vi "探头通信模块.vi"(11 "探头属性":T8={"探头地址与信息"={"网络地址"="四渡赤水", "名称"="四渡赤水", "备注"="10.10.100.254", "累积剂量"=8899.0, "累积限值"=0.0, "硬件剂量率限值"=enum."一级限值", "剂量率限值1"=0.0, "剂量率限值2"=0.0, "报警方式"=enum."常报警"}, "测量值"={"时间"=timestamp(0 s since 1904-01-01), "数值"=0.0}, "限值"={"限值1"=1.0, "限值2"=100.0, "探头限值"=enum."一级限值"}, "探头状态"=enum."离线", "累积记录"={"起始时间"=timestamp(0 s since 1904-01-01), "结束时间"=timestamp(0 s since 1904-01-01), "累积剂量"=0.0}, "报警方式"={"报警方式"=enum."常报警", "延迟计时"=0, "报警中？"=FALSE}}) -> ()   [LabVIEW 2017]
doc: "独立的探头TCP连接的接收处理模块，具有\"创建TCP连接\"，“自动同步报警限值”，“掉线重连”，“解析实时数据与报警数据”的功能。"
uses:
  <vilib>/Platform/TimedLoop/XDataNode/timing_clust.ctl
  <vilib>/Platform/TimedLoop/XDataNode/nitl_modes.ctl
  <vilib>/Platform/TimedLoop/XDataNode/wakeup.ctl
  0d55e998-beb3-44e2-a108-1cc669182013.vi
  <vilib>/regexp/Match Regular Expression.xnode
  <vilib>/Platform/TimedLoop/XDataNode/XDataNode.xnode
  <vilib>/Platform/TimedLoop/XDataNode/XDNodeRunTimeDep.lvlib
panel:
  in  "报警缓存防抖计次":i32
  in  "串口丢包次数":i32
  out "接收数据":string
  out "循环次数":i32
  out "TCP连接ID":refnum<k5>
  in  "通信错误":errorcluster caption="错误输出"
  in  "缓存结果":T1
  in  "改动项":T3
  in  "停止":bool
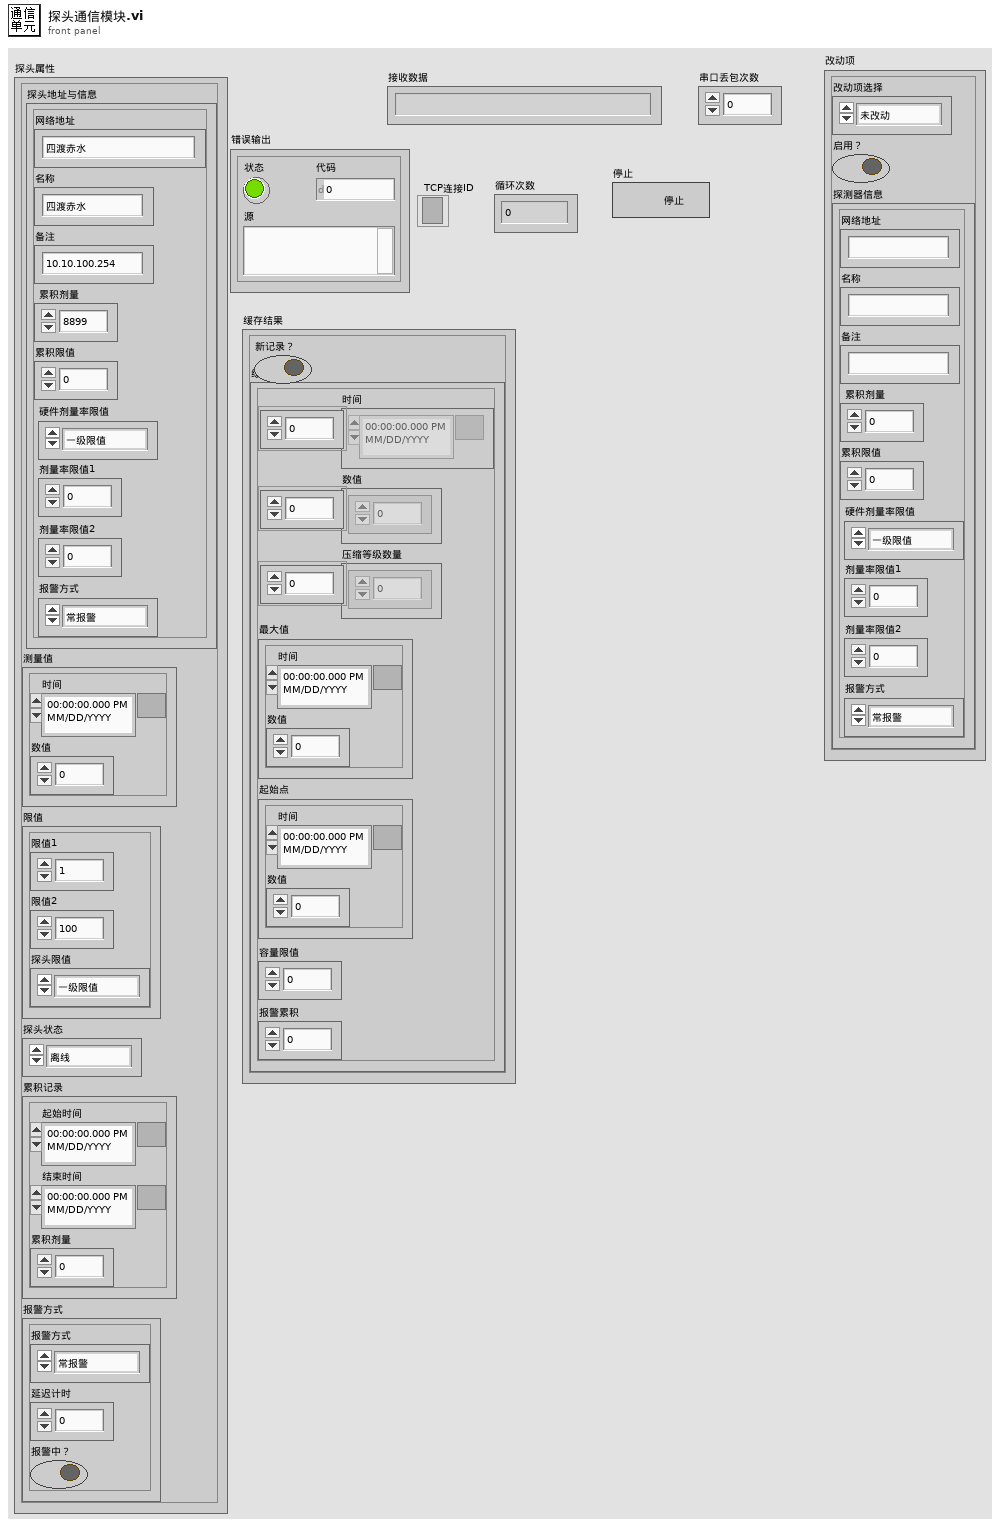
[diagram p1: front panel]
types:
  T1 = typedef "报警缓存状态与数据.ctl" = cluster{"新记录？":bool, "缓存数据":T2}
  T2 = typedef "时值缓存压缩模块.lvlib/缓存数据.ctl" = cluster{"时间":timestamp[], "数值":dbl[], "压缩等级数量":i32[], "最大值":cluster{"时间":timestamp, "数值":dbl}, "起始点":cluster{"时间":timestamp, "数值":dbl}, "容量限值":i32, "报警累积":dbl}
  T3 = typedef "改动项.ctl" = cluster{"改动项选择":T4, "启用？":bool, "探测器信息":T5}
  T4 = typedef "改动项选择.ctl" = enum16{"未改动", "改动-启用状态", "改动-探头信息", "改动-报警限值", "动作-手动静音", "动作-重启累积时段", "动作-累积删除", "动作-重连"}
  T5 = typedef "探测器信息.ctl" = cluster{"网络地址":string, "名称":string, "备注":string, "累积剂量":dbl, "累积限值":dbl, "硬件剂量率限值":T6, "剂量率限值1":dbl, "剂量率限值2":dbl, "报警方式":T7}
  T6 = typedef "探头剂量率限值选择.ctl" = enum16{"一级限值", "二级限值"}
  T7 = typedef "报警方式选择.ctl" = enum16{"常报警", "自动静音", "手动静音"}
  T8 = typedef "探头属性.ctl" = cluster{"探头地址与信息":T5, "测量值":T9, "限值":T10, "探头状态":T11, "累积记录":T12, "报警方式":T13}
  T9 = typedef "测量值.ctl" = cluster{"时间":timestamp, "数值":dbl}
  T10 = typedef "剂量率限值.ctl" = cluster{"限值1":dbl, "限值2":dbl, "探头限值":T6}
  T11 = typedef "探头状态.ctl" = enum16{"正常", "离线", "禁用", "一级报警", "二级报警", "累积报警"}
  T12 = typedef "单条累积记录.ctl" = cluster{"起始时间":timestamp, "结束时间":timestamp, "累积剂量":dbl}
  T13 = typedef "报警方式.ctl" = cluster{"报警方式":T7, "延迟计时":u16, "报警中？":bool}
  T14 = typedef "簇-输入.ctl" = cluster{"配置文件动作":T15, "数据输入":variant}
  T15 = typedef "枚举-配置文件动作.ctl" = enum16{"初始化加载配置", "读取配置", "写入-屏幕键盘", "写入-静音延迟", "写入-主要探头类型", "写入-串口配置", "写入-累积定时", "写入-导出定时", "保存配置到文件"}
  T16 = typedef "簇-配置文件内容.ctl" = cluster{"调试模式？":bool, "屏幕键盘？":bool, "软件版本":string, "静音延迟 s":u16, "主要探头类型":T17, "串口配置":cluster{"COM口":refnum<visa-resource-name>, "波特率":enum16{"9600", "19200"}, "读写超时ms":i16, "丢包判定次数":i16}, "定时配置-累积分段":T18, "定时配置-自动导出":cluster{"定时配置-自动导出":T18, "分别导出?":bool}}
  T17 = typedef "枚举-主要探头类型.ctl" = enum16{"网络探头", "串口探头"}
  T18 = typedef "簇-定时配置.ctl" = cluster{"定时模式":enum16{"绝对时间", "相对时间"}, "单位":enum16{"年", "月", "日", "时", "分"}, "间隔":u8, "目标时刻":timestamp}
  T19 = typedef "串口配置.ctl" = cluster{"COM口":refnum<visa-resource-name>, "波特率":enum16{"9600", "19200"}, "探头地址(U8)":u8}
  T20 = typedef "串口模块输入.ctl" = cluster{"串口动作类型":T21, "串口配置":T19, "数据输入":variant}
  T21 = typedef "串口动作类型.ctl" = enum16{"读测量值", "设置报警值", "设置地址", "设置系数", "广播修改波特率", "关闭串口"}
  T22 = typedef "DB动作与数据.ctl" = cluster{"动作类型":T23, "输入数据":variant}
  T23 = typedef "DB动作类型.ctl" = enum16{"DB-文件初始化+连接", "DB-断开连接", "DB-结构初始化", "DB-加载设备", "DB-检查连接状态", "设备-登记新设备+数据表", "设备-删除设备", "设备-修改网址", "设备-修改名称+转移数据", "设备-修改备注", "设备-修改限值", "设备-累积校准", "设备-重排", "数据-获取全部", "数据-删除数据", "数据-写改累积记录+改累积剂量", "读变量-全部设备"}
  T24 = typedef "测量值读取.ctl" = cluster{"测量值":dbl, "CRC":bool, "接收指令":string}
  T25 = typedef "写改累积记录输入.ctl" = cluster{"探头地址与信息":T5, "测量值":T9, "累积记录":T12}
  T26 = cluster{"报警方式":enum16{"常报警", "自动静音", "手动静音"}, "延迟计时":u16, "报警中？":bool}
  T27 = typedef "XDNodeRunTimeDep.lvlib/timing_clust.ctl" = cluster{"Expected End [f-1]":u64, "Actual End [f-1]":u64, "Finished Late? [f-1]":bool, "Expected End [i-1]":u64, "Actual End [i-1]":u64, "Finished Late? [i-1]":bool, "Expected Start [i]":u64, "Actual Start [i]":u64, "Expected Start [f]":u64, "Actual Start [f]":u64, "Source Name":string, "Structure Name":string, "Period":i64, "Deadline":i64, "Offset":i64, "Start":i64, "Priority":i32, "Timeout":i32, "Mode":T28, "Wakeup Reason":T29, "Error":errorcluster, "Source Type":string, "Secondary Source Type":string, "Global End Time":u64, "Global Start Time":u64, "Frame Duration":u64, "Iteration Duration":u64, "Assigned CPU":i32, "I/O Scan Engine Mode":u32}
  T28 = typedef "XDNodeRunTimeDep.lvlib/nitl_modes.ctl" = enum32{"No Change", "Process missed periods, maintain original phase", "Discard missed periods, maintain original phase", "Process missed periods, ignore original phase", "Discard missed periods, ignore original phase"}
  T29 = typedef "XDNodeRunTimeDep.lvlib/wakeup.ctl" = enum32{"Normal", "Aborted", "Asynchronous wakeup", "Timing source error", "Timed loop error", "Timeout"}
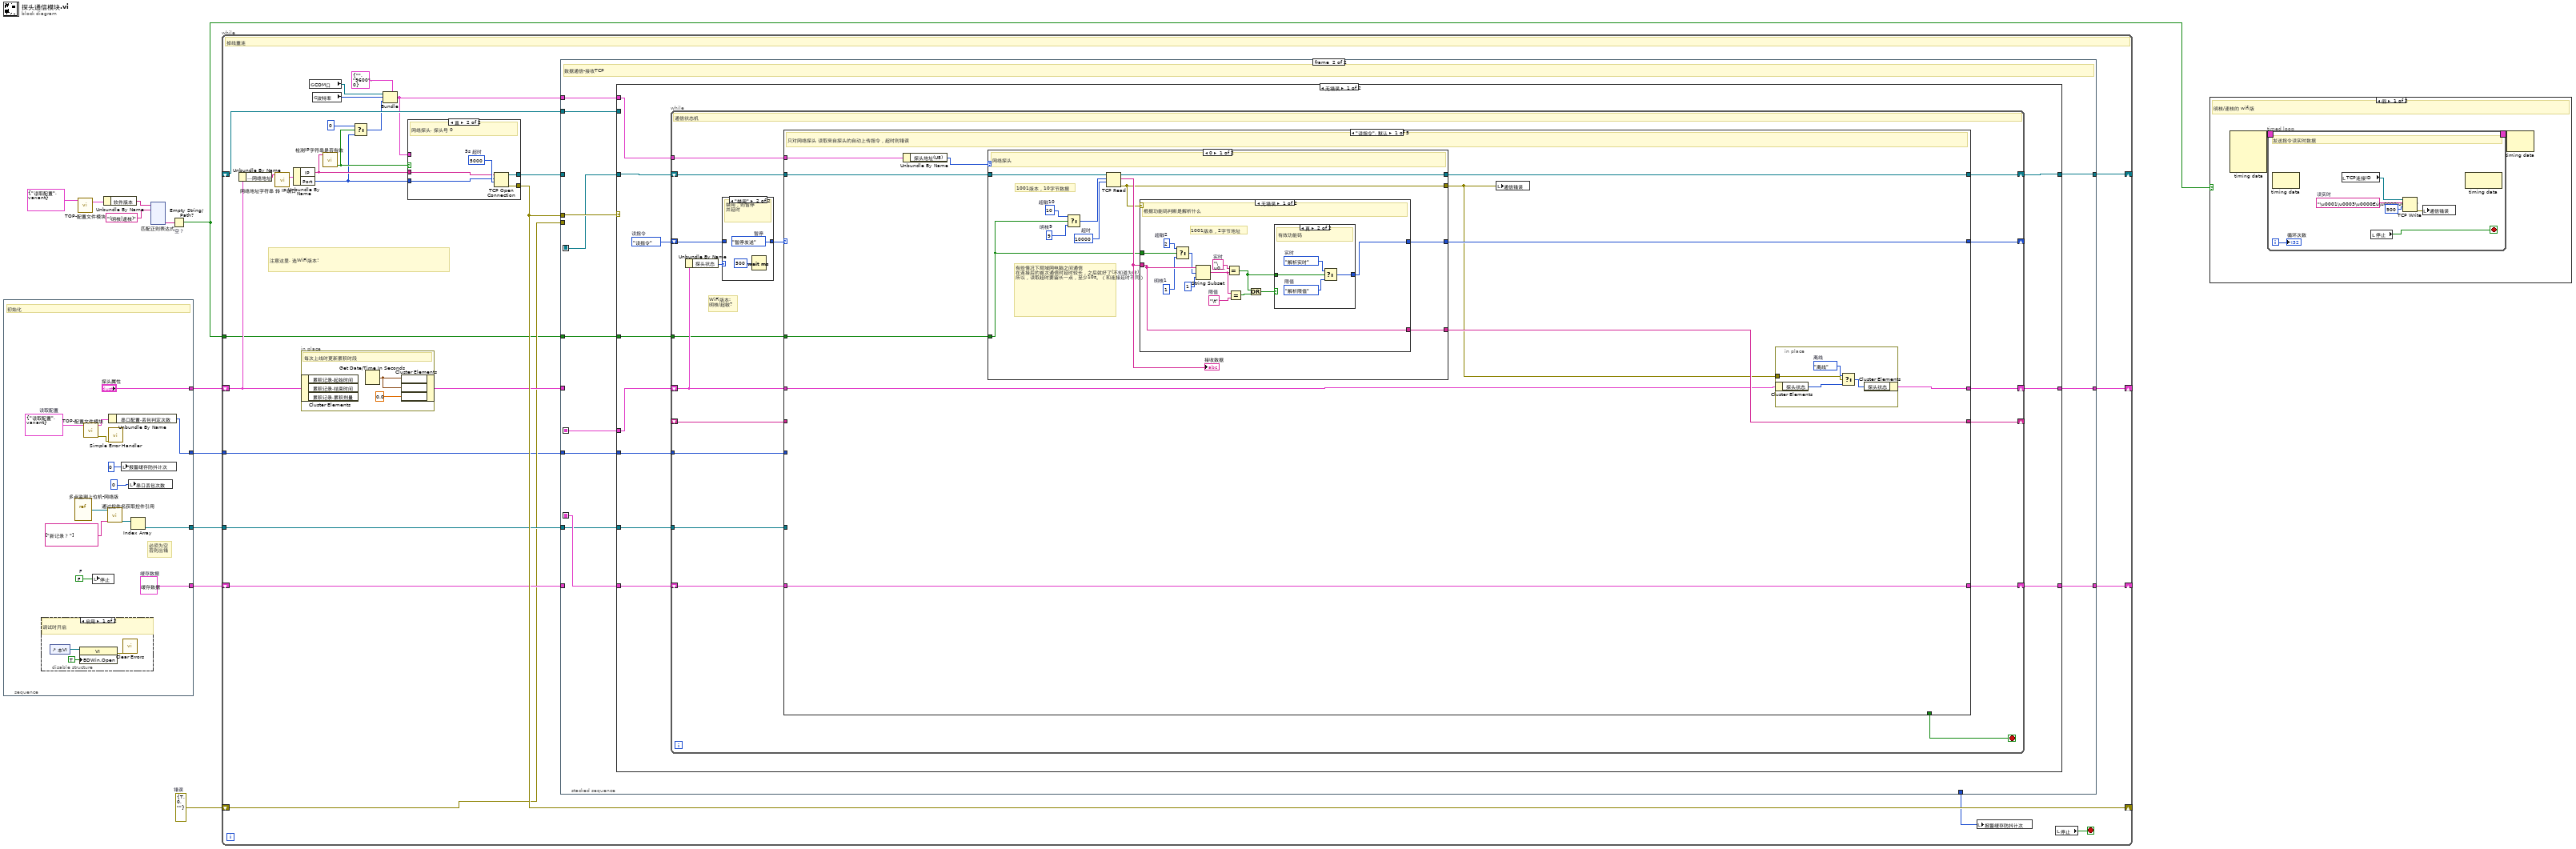
[diagram p0: block diagram]
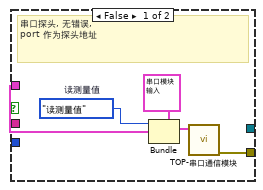
[diagram p4: hidden frame]
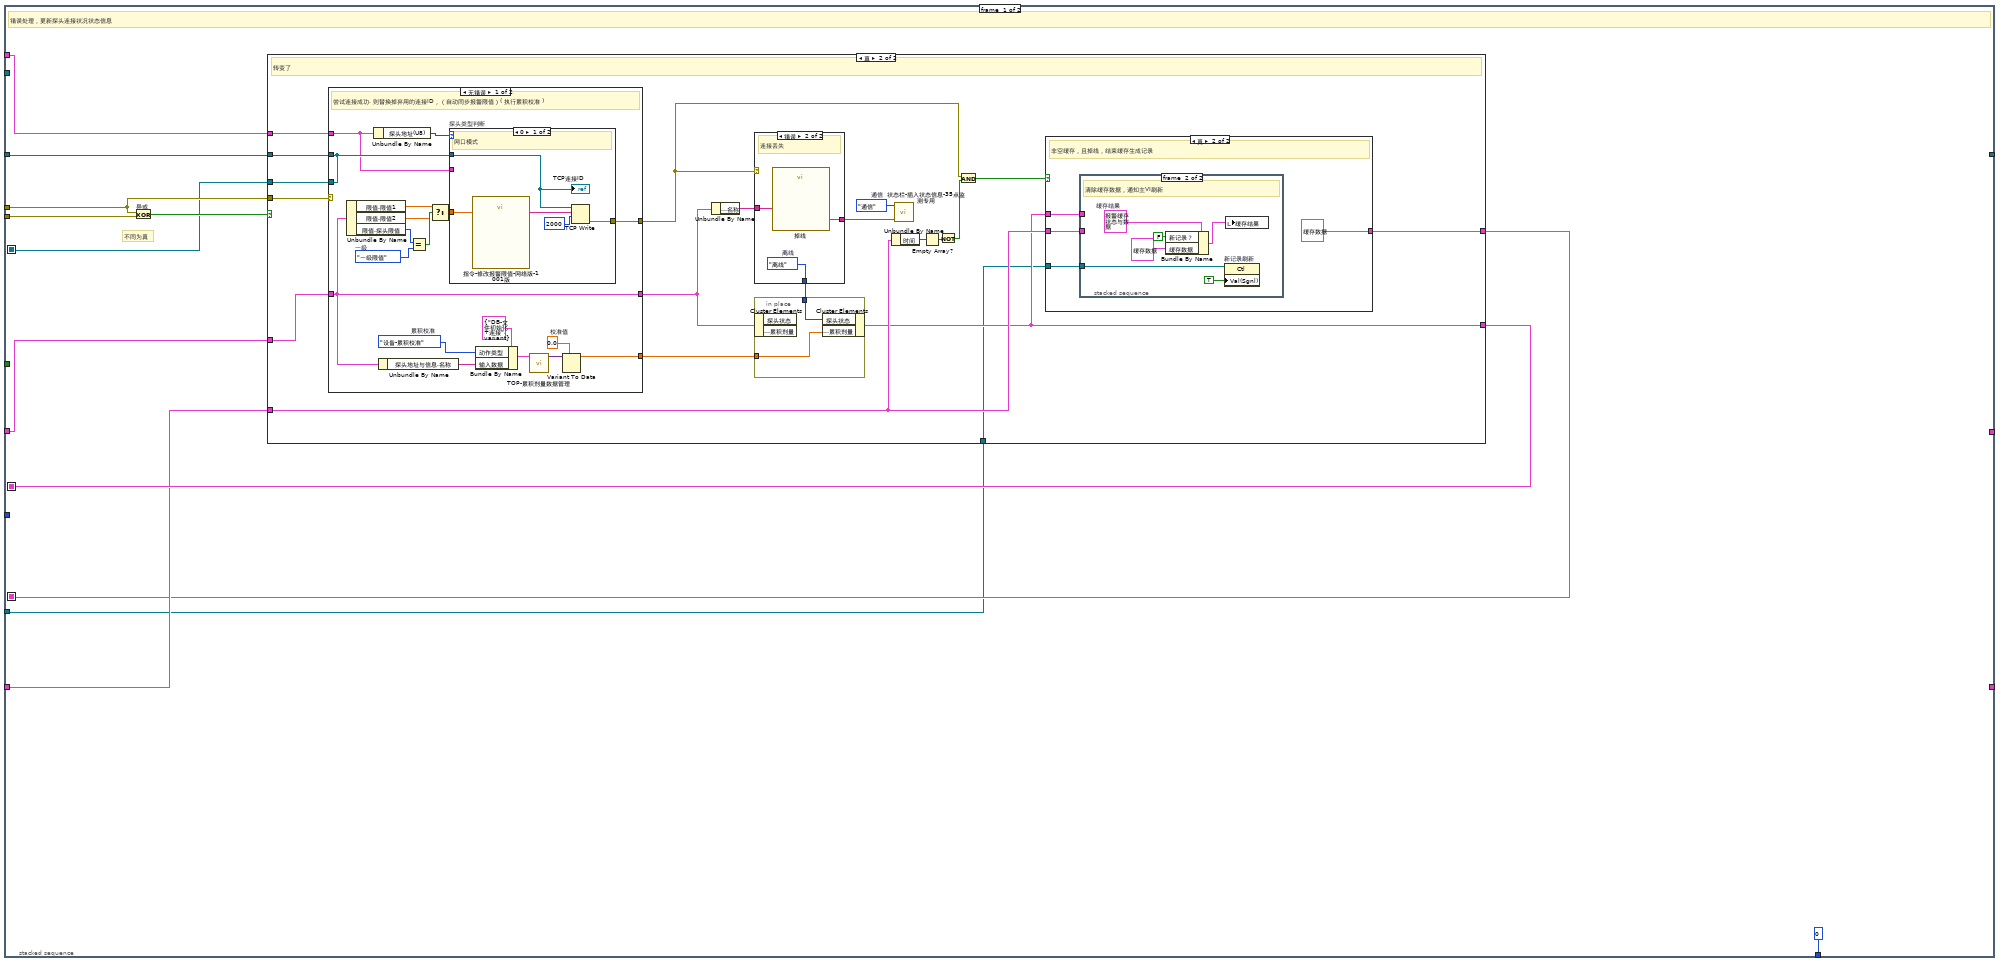
[diagram p5: hidden frame]
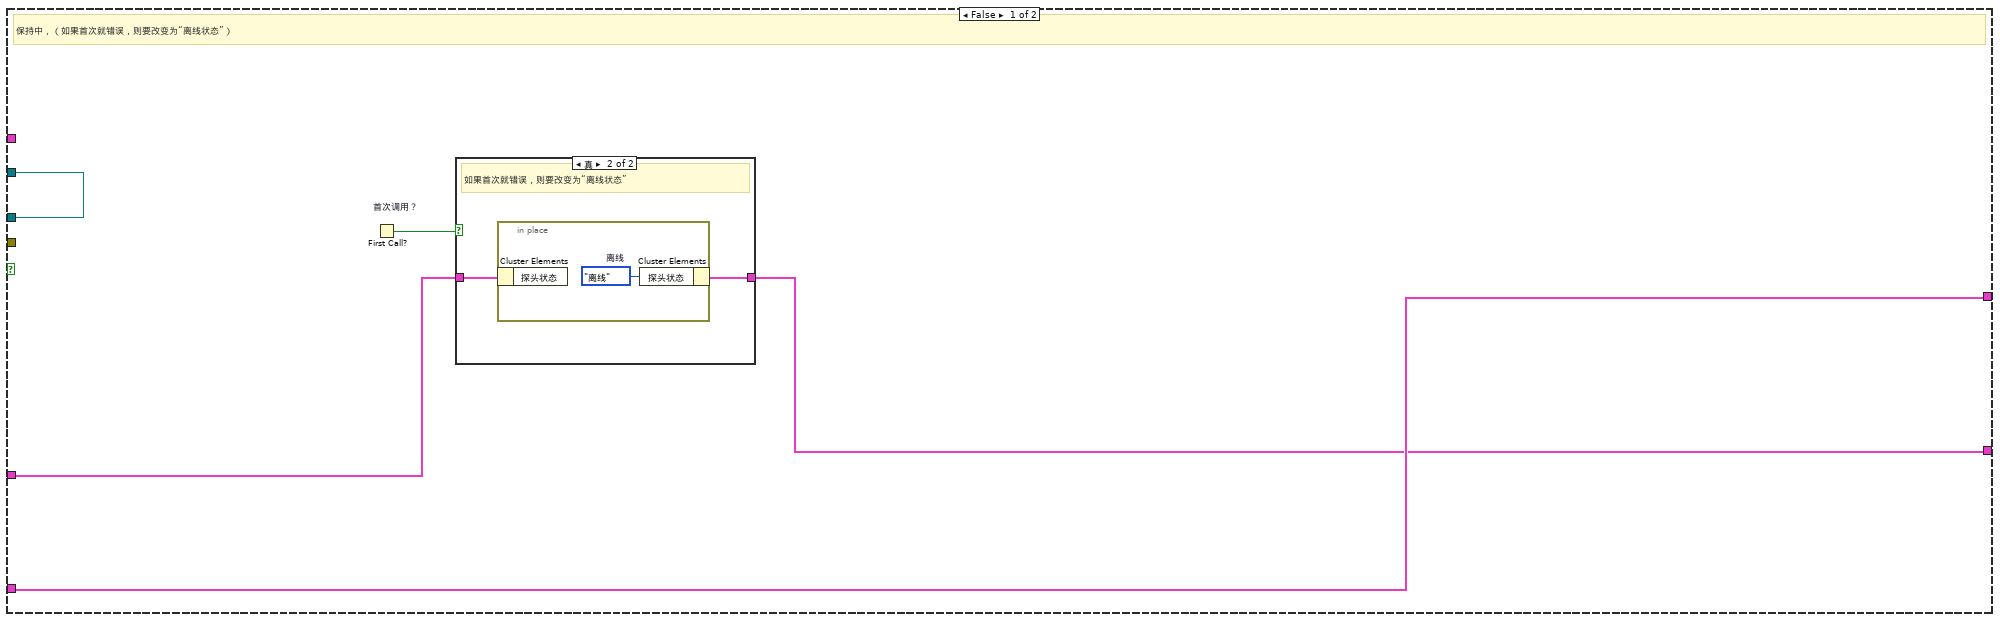
[diagram p6: hidden frame]
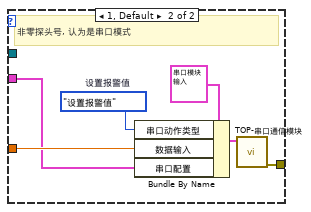
[diagram p8: hidden frame]
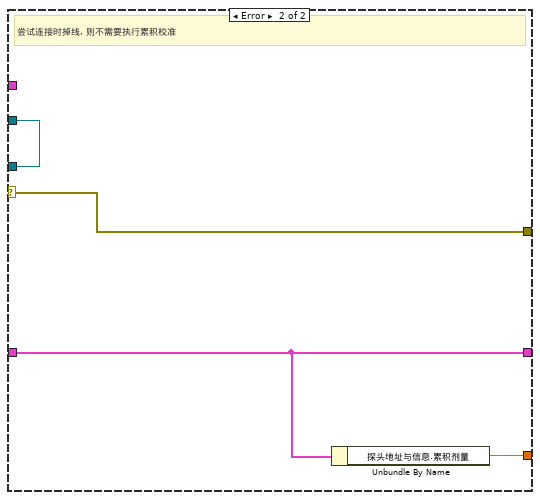
[diagram p9: hidden frame]
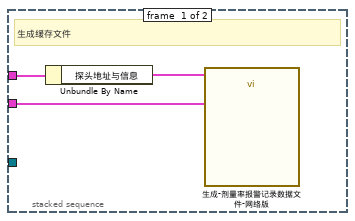
[diagram p11: hidden frame]
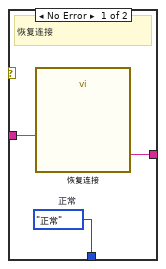
[diagram p12: hidden frame]
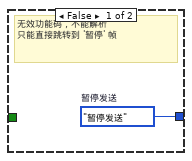
[diagram p14: hidden frame]
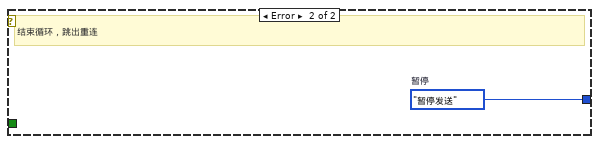
[diagram p15: hidden frame]
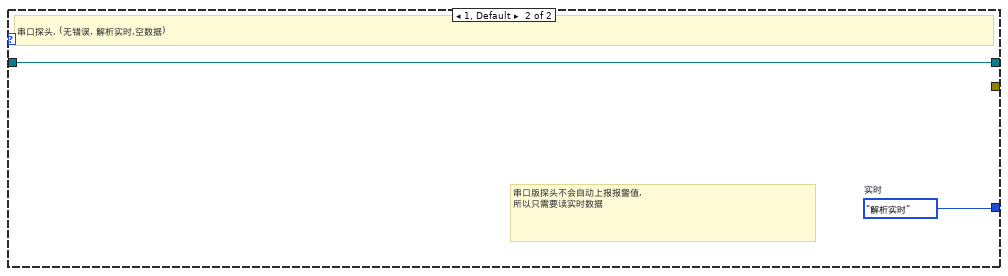
[diagram p16: hidden frame]
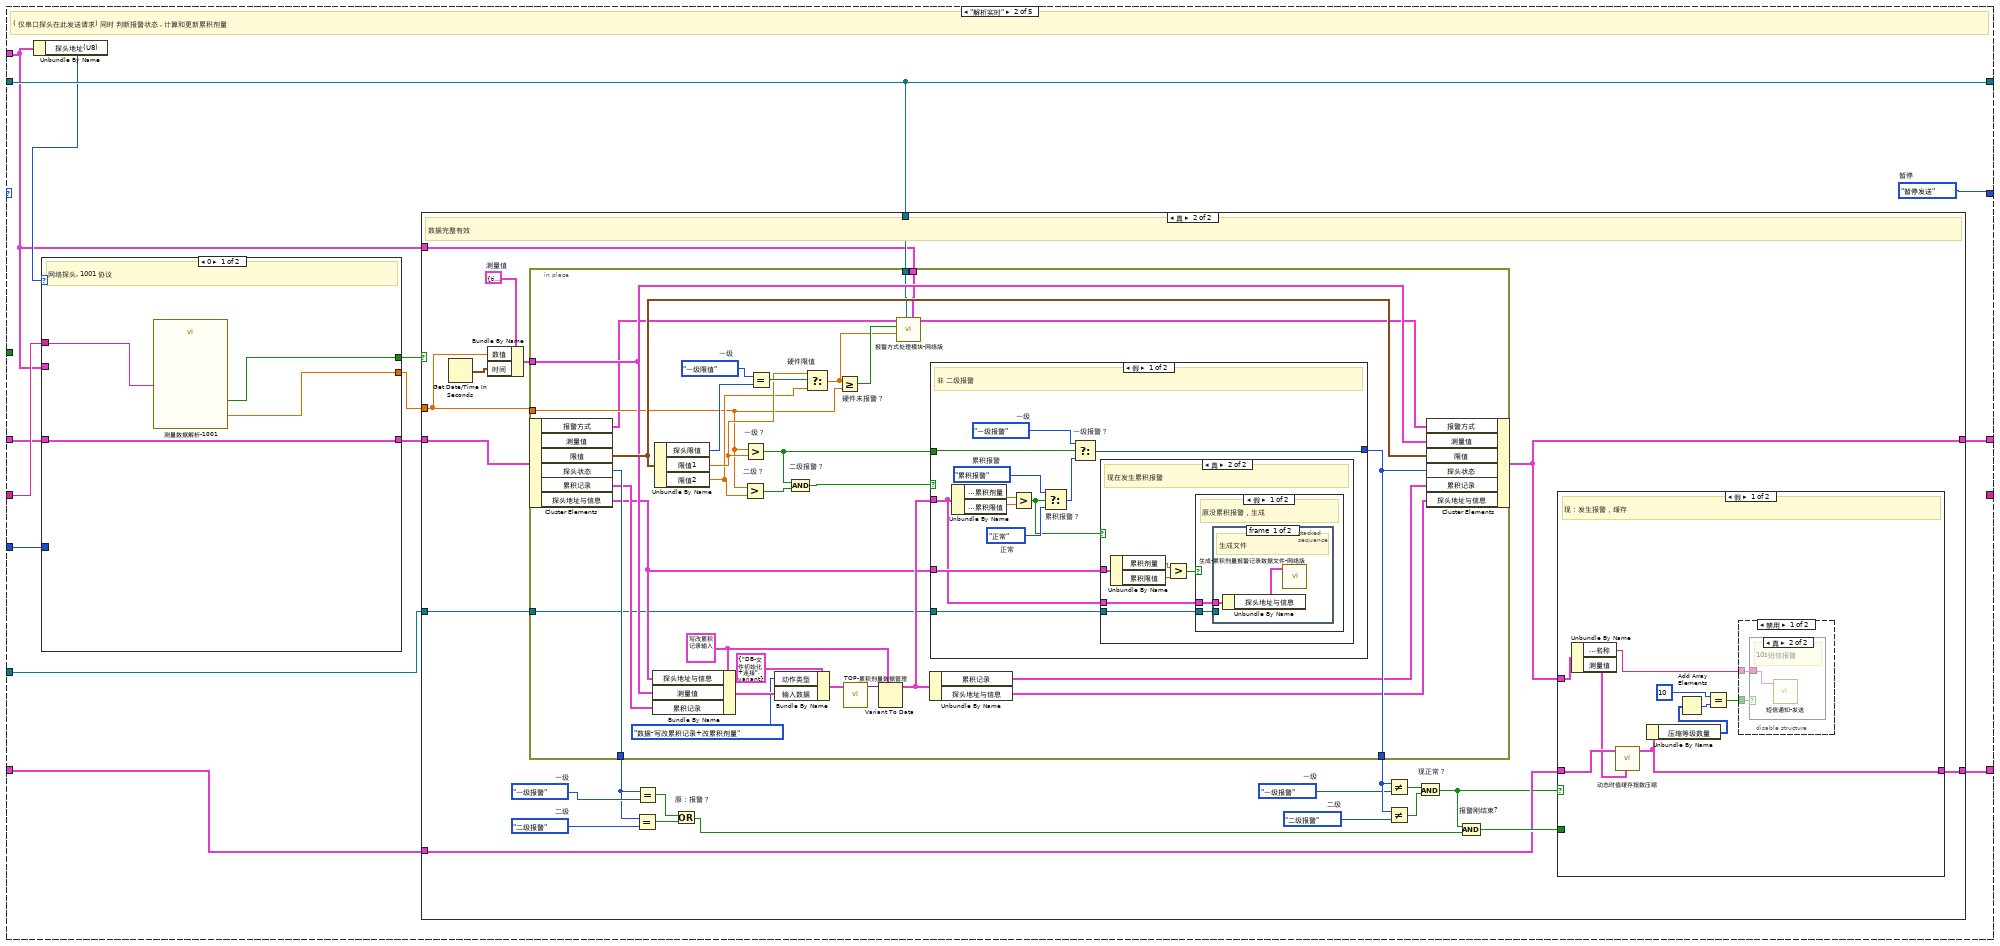
[diagram p17: hidden frame]
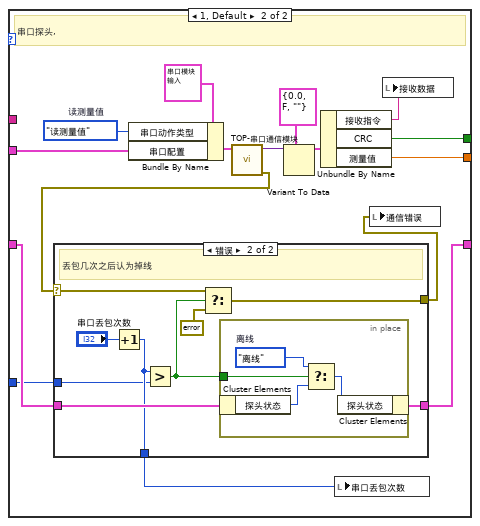
[diagram p18: hidden frame]
diagram:
  w11 = errorcluster {"status"=TRUE, "code"=0, "source"=""}  # 错误
  n1 = stacked-sequence {
    tunnel: ["探头属性"] -> w10
    tunnel: [w19] -> w9
    tunnel: [w20] -> w8
    tunnel: [w12] -> w7
    frame #0 {
      w15 = T14 {"配置文件动作"=enum."读取配置", "数据输入"=variant}  # 读取配置
      w19 = T2 {"时间"=[], "数值"=[], "压缩等级数量"=[], "最大值"={"时间"=timestamp(0 s since 1904-01-01), "数值"=0.0}, "起始点"={"时间"=timestamp(0 s since 1904-01-01), "数值"=0.0}, "容量限值"=0, "报警累积"=0.0}  # 缓存数据
      w24 = FALSE  # F
      # "必须为空\n否则出错"
      # "初始化"
      n2 = disable-structure shown="启用" {
        frame Enabled {
          # "调试时开启"
          n3 = control-ref of="本VI"() -> (w27:refnum<vi>)
          n4 = property class="VI"(reference=w27, "BDWin.Open"=TRUE ("程序框图窗口:打开")) -> (error out=w25:errorcluster)  [unwired: 1 in, 1 out]
          n5 = call <vilib>:"Clear Errors.vi"("error in (no error)"=w25) -> ()  [unwired: 5 in, 2 out]
        }
        frame Disabled {
        }
      }
      n6 = vi-ref "多点监测上位机-网络版.vi"() -> (w23:refnum<vi>)
      n7 = call "TOP-配置文件模块.vi"("输入"=w15) -> ("error out"=w14:errorcluster, "配置文件"=w13:T16)  [unwired: 9 in]
      n8 = local write "停止"(w24) -> ()
      n9 = call "通过控件名获取控件引用.vi"("控件名数组"=string[] ["新记录？"], "VI引用"=w23) -> ("控件引用输出"=w21:refnum<vi>[])  [unwired: 7 in, 2 out]
      n10 = Unbundle By Name(w13) -> ("串口配置.丢包判定次数"=w12:i16)
      n11 = call <vilib>:"Simple Error Handler.vi"("error in (no error)"=w14) -> ()  [unwired: 4 in, 5 out]
      n12 = local write "报警缓存防抖计次"(0 ("数值输入控件")) -> ()
      n13 = local write "串口丢包次数"(0 ("串口丢包次数")) -> ()
      n14 = Index Array(array=w21) -> (element=w20:refnum<vi>)  [unwired: 1 in]
    }
  }
  n15 = call "TOP-配置文件模块.vi"("输入"=T14 {"配置文件动作"=enum."读取配置", "数据输入"=variant}) -> ("配置文件"=w4:T16)  [unwired: 9 in, 1 out]
  n16 = Unbundle By Name(w4) -> ("软件版本"=w5:string)
  n17 = xnode "匹配正则表达式"("输入字符串"=w5, "正则表达式"="(明核|速核)") -> ("子匹配 1"=w6:string)  [unwired: 4 in, 5 out]
  n18 = Empty String/Path? "空？"(string/path=w6) -> (empty?=w1:bool)
  n19 = while {
    shift-right: [w52] -> _
    shift-left: w11 -> [w40]
    shift-right: [w53] -> _
    shift-left: w10 -> [w42]
    shift-right: [w49] -> _
    shift-left: w9 -> [w51]
    shift-right: [w48] -> _
    shift-left: _ -> [w47]
    tunnel: w8 -> [w44]
    tunnel: w7 -> [w29]
    tunnel: w1 -> [w28]
    stop <- w45 stop-if-true
    # "注意这里, 选WiFi版本!"
    # "掉线重连"
    n20 = Unbundle By Name(w42) -> ("探头地址与信息.网络地址"=w50:string)
    n21 = call "网络地址字符串 转 IP端口.vi"("IP端口字符串"=w50) -> ("IP端口"=w43:cluster{"IP":string, "Port":u16})  [unwired: 10 in]
    n22 = Unbundle By Name(w43) -> ("IP"=w39:string, "Port"=w33:u16)
    n23 = in-place {
      # "每次上线时更新累积时段"
      n24 = in-place-cluster #1(w42) -> ()  [unwired: 3 out]
      n25 = Get Date/Time In Seconds() -> (seconds since 1Jan1904=w65:timestamp)
      n26 = in-place-cluster #1("累积记录.起始时间"=w65, "累积记录.结束时间"=w65, "累积记录.累积剂量"=0.0) -> (w41:T8)
    }
    n27 = global read "全局变量-35点监测.vi" "COM口"() -> (w36:refnum<visa-resource-name>)
    n28 = global read "全局变量-35点监测.vi" "波特率"() -> (w37:enum16{"9600", "19200"})
    n29 = call "检测IP字符串是否有效.vi"("IP地址"=w39) -> ("有效IP？"=w35:bool)  [unwired: 10 in]
    n30 = Select(t=0, s=w35, f=w33) -> (s? t:f=w32:i32)
    n31 = Bundle(cluster=T19 {"COM口"="", "波特率"=enum."9600", "探头地址(U8)"=0} ("串口配置"), "COM口"=w36, "波特率"=w37, "探头地址(U8)"=w32) -> (w31:T19)
    n32 = case shown="真" w35 {
      tunnel: [w54 w62] -> w52
      tunnel: [_ w61] -> w46
      tunnel: w33 -> [_ w60]
      tunnel: w39 -> [_ w59]
      tunnel: w31 -> [w55 _]
      frame False {
        w56 = 串口动作类型."读测量值"  # 读测量值
        # "串口探头, 无错误,\nport 作为探头地址"
        n33 = Bundle(cluster=T20 {"串口动作类型"=enum."读测量值", "串口配置"={"COM口"="", "波特率"=enum."9600", "探头地址(U8)"=0}, "数据输入"=variant} ("串口模块输入"), "串口动作类型"=w56, "串口配置"=w55) -> (w58:T20)  [unwired: 1 in]
        n34 = call "TOP-串口通信模块.vi"("串口模块输入"=w58) -> ("error out"=w54:errorcluster)  [unwired: 9 in, 1 out]
      }
      frame True {
        w63 = 5000  # 5s 超时
        # "网络探头, 探头号 0"
        n35 = TCP Open Connection(address=w59, remote port or service name=w60, timeout ms (60000)=w63) -> (connection ID=w61:refnum<k5>, error out=w62:errorcluster)  [unwired: 2 in]
      }
    }
    n36 = stacked-sequence {
      seq-local: [w74 _] -> [_ w171]
      seq-local: [w72 _] -> [_ w169]
      seq-local: [w71 _] -> [_ w167]
      tunnel: w46 -> [w70 _]
      tunnel: w52 -> [w76 w173]
      tunnel: w40 -> [w77 _]
      tunnel: w41 -> [w68 _]
      tunnel: [_ w172] -> w53
      tunnel: w51 -> [w73 _]
      tunnel: [_ w170] -> w49
      tunnel: [_ w168] -> w48
      tunnel: w47 -> [_ w166]
      tunnel: w44 -> [w67 w165]
      tunnel: w31 -> [w69 w164]
      tunnel: [0 ("报警缓存防抖计次") _] -> w30
      tunnel: w29 -> [_ w163]
      tunnel: w28 -> [_ w162]
      frame #0 {
        # "不同为真"
        # "错误处理，更新探头连接状况状态信息"
        n37 = Exclusive Or "异或"(1:w77, 2:w76) -> (0:w75:bool)
        n38 = case shown="真" w75 {
          tunnel: w76 -> [_ w95]
          tunnel: w68 -> [w80 w91]
          tunnel: [w79 w88] -> w74
          tunnel: w73 -> [w82 w93]
          tunnel: [w82 w98] -> w72
          tunnel: w70 -> [w81 w97]
          tunnel: [w81 w96] -> w71
          tunnel: w69 -> [_ w92]
          tunnel: w67 -> [_ w87]
          frame False {
            # "保持中，（如果首次就错误，则要改变为“离线状态”）"
            n39 = First Call? "首次调用？"() -> (First Call?: T/F=w78:bool)
            n40 = case shown="真" w78 {
              tunnel: w80 -> [w83 w85]
              tunnel: [w83 w84] -> w79
              frame False {
                # "非首次"
              }
              frame True {
                # "如果首次就错误，则要改变为“离线状态”"
                n41 = in-place {
                  w86 = 探头状态."离线"  # 离线
                  n42 = in-place-cluster #2(w85) -> ()  [unwired: 1 out]
                  n43 = in-place-cluster #2("探头状态"=w86) -> (w84:T8)
                }
              }
            }
          }
          frame True {
            w106 = enum16{"全部", "报警", "通信", "设置"}."通信"  # 通信
            # "转变了"
            n44 = case shown="无错误" w95 {
              selector: w95 -> [_ w139]
              tunnel: w97 -> [w117 w138]
              tunnel: w91 -> [w108 w137]
              tunnel: [w117 w138] -> w96
              tunnel: [w124 w139] -> w94
              tunnel: w92 -> [w115 _]
              tunnel: [w108 w137] -> w90
              tunnel: [w107 w136] -> w89
              frame No Error {
                w111 = 0.0  # 校准值
                w109 = DB动作类型."设备-累积校准"  # 累积校准
                w122 = enum16{"一级限值", "二级限值"}."一级限值"  # 一级
                # "尝试连接成功, 则替换掉弃用的连接ID，（自动同步报警限值）( 执行累积校准 )"
                n45 = Unbundle By Name(w108) -> ("限值.限值1"=w119:dbl, "限值.限值2"=w120:dbl, "限值.探头限值"=w123:T6)
                n46 = Unbundle By Name(w115) -> ("探头地址(U8)"=w116:u8)
                n47 = Unbundle By Name(w108) -> ("探头地址与信息.名称"=w113:string)
                n48 = Equal?(x=w123, y=w122) -> (x = y?=w121:bool)
                n49 = Select(t=w119, s=w121, f=w120) -> (s? t:f=w118:dbl)
                n50 = case "探头类型判断" shown="0" w116 {
                  tunnel: [w129 w135] -> w124
                  tunnel: w118 -> [w126 w131]
                  tunnel: w117 -> [w125 _]
                  tunnel: w115 -> [_ w130]
                  frame 0 {
                    # "网口模式"
                    n51 = call "指令-修改报警限值-网络版-1001版.vi"("限值"=w126) -> ("指令输出"=w128:string)  [unwired: 10 in]
                    n52 = TCP Write(connection ID=w125, data in=w128, 9:2000 ("超时毫秒(25000)")) -> (error out=w129:errorcluster)  [unwired: 1 in, 2 out]
                    "TCP连接ID" <- w125
                  }
                  frame 1, Default {
                    w132 = 串口动作类型."设置报警值"  # 设置报警值
                    # "非零探头号, 认为是串口模式"
                    n53 = Bundle By Name(cluster=T20 {"串口动作类型"=enum."读测量值", "串口配置"={"COM口"="", "波特率"=enum."9600", "探头地址(U8)"=0}, "数据输入"=variant} ("串口模块输入"), "串口动作类型"=w132, "数据输入"=w131, "串口配置"=w130) -> (w133:T20)
                    n54 = call "TOP-串口通信模块.vi"("串口模块输入"=w133) -> ("error out"=w135:errorcluster)  [unwired: 9 in, 1 out]
                  }
                }
                n55 = Bundle By Name(cluster=T22 {"动作类型"=enum."DB-文件初始化+连接", "输入数据"=variant} ("DB动作集"), "动作类型"=w109, "输入数据"=w113) -> (w112:T22)
                n56 = call "TOP-累积剂量数据管理.vi"("DB动作集"=w112) -> ("输出数据"=w114:variant)  [unwired: 9 in, 1 out]
                n57 = Variant To Data(type=w111, Variant=w114) -> (data=w107:dbl)  [unwired: 1 in, 1 out]
              }
              frame Error {
                # "尝试连接时掉线, 则不需要执行累积校准"
                n58 = Unbundle By Name(w137) -> ("探头地址与信息.累积剂量"=w136:dbl)
              }
            }
            n59 = Unbundle By Name(w90) -> ("探头地址与信息.名称"=w104:string)
            n60 = case "生成" shown="错误" w94 {
              tunnel: [w157 w161] -> w105
              tunnel: w104 -> [w158 w160]
              tunnel: [w156 w159] -> w103
              frame No Error {
                w156 = 探头状态."正常"  # 正常
                # "恢复连接"
                n61 = call "恢复连接"("探头信息"=w158) -> ("Result"=w157:string)  [unwired: 13 in, 1 out]
              }
              frame Error {
                w159 = 探头状态."离线"  # 离线
                # "连接丢失"
                n62 = call "掉线"("探头信息"=w160) -> ("Result"=w161:string)  [unwired: 13 in, 1 out]
              }
            }
            n63 = in-place {
              in-place-border: w103 -> [w155]
              in-place-border: w89 -> [w154]
              n64 = in-place-cluster #3(w90) -> ()  [unwired: 2 out]
              n65 = in-place-cluster #3("探头状态"=w155, "探头地址与信息.累积剂量"=w154) -> (w88:T8)
            }
            n66 = Unbundle By Name(w93) -> ("时间"=w102:timestamp[])
            n67 = call "状态栏-插入状态信息-35点监测专用.vi"("消息内容"=w105, "状态类型"=w106) -> ()  [unwired: 10 in]
            n68 = Empty Array?(array=w102) -> (empty?=w101:bool)
            n69 = Not(x=w101) -> (.not. x?=w100:bool)
            n70 = And(x=w94, y=w100) -> (x .and. y?=w99:bool)
            n71 = case shown="真" w99 {
              tunnel: w93 -> [w140 w142]
              tunnel: [w140 T2 {"时间"=[], "数值"=[], "压缩等级数量"=[], "最大值"={"时间"=timestamp(0 s since 1904-01-01), "数值"=0.0}, "起始点"={"时间"=timestamp(0 s since 1904-01-01), "数值"=0.0}, "容量限值"=0, "报警累积"=0.0} ("缓存数据")] -> w98
              tunnel: w88 -> [_ w143]
              tunnel: w87 -> [_ w141]
              frame False {
                # "没有在缓存的数据"
              }
              frame True {
                # "非空缓存，且掉线，结束缓存生成记录"
                n72 = stacked-sequence {
                  tunnel: w142 -> [w147 _]
                  tunnel: w143 -> [w146 _]
                  tunnel: w141 -> [_ w153]
                  frame #0 {
                    # "生成缓存文件"
                    n73 = Unbundle By Name(w146) -> ("探头地址与信息"=w145:T5)
                    n74 = call "生成-剂量率报警记录数据文件-网络版.vi"("缓存绘图数据"=w147, "探测器信息"=w145) -> ()  [unwired: 10 in]
                  }
                  frame #1 {
                    w150 = T1 {"新记录？"=FALSE, "缓存数据"={"时间"=[], "数值"=[], "压缩等级数量"=[], "最大值"={"时间"=timestamp(0 s since 1904-01-01), "数值"=0.0}, "起始点"={"时间"=timestamp(0 s since 1904-01-01), "数值"=0.0}, "容量限值"=0, "报警累积"=0.0}}  # 缓存结果
                    # "清除缓存数据，通知主VI刷新"
                    n75 = Bundle By Name(cluster=w150, "新记录？"=FALSE, "缓存数据"=T2 {"时间"=[], "数值"=[], "压缩等级数量"=[], "最大值"={"时间"=timestamp(0 s since 1904-01-01), "数值"=0.0}, "起始点"={"时间"=timestamp(0 s since 1904-01-01), "数值"=0.0}, "容量限值"=0, "报警累积"=0.0}) -> (w151:T1)
                    n76 = property on="新记录刷新" class="Ctl"(reference=w153, "Val(Sgnl)"=TRUE) -> ()  [unwired: 1 in, 2 out]
                    n77 = local write "缓存结果"(w151) -> ()
                  }
                }
              }
            }
          }
        }
      }
      frame #1 {
        # "数据通信-接收TCP"
        n78 = case shown="无错误" w173 {
          tunnel: w171 -> [w183 w513]
          tunnel: [w182 w512] -> w172
          tunnel: w169 -> [w181 w520]
          tunnel: [w180 w520] -> w170
          tunnel: [w179 w518] -> w168
          tunnel: w167 -> [w178 _]
          tunnel: w166 -> [_ w515]
          tunnel: w165 -> [w177 _]
          tunnel: w164 -> [w176 w511]
          tunnel: w163 -> [w175 _]
          tunnel: w162 -> [w174 _]
          frame No Error {
            w184 = enum16{"读指令", "解析实时", "解析限值", "暂停发送", "读取超时"}."读指令"  # 读指令
            n79 = while {
              shift-right: [w199] -> _
              shift-left: w184 -> [w191]
              shift-right: [w200] -> w179
              shift-left: w178 -> [w201]
              shift-right: [w197] -> _
              shift-left: _ -> [w196]
              shift-right: [w195] -> w182
              shift-left: w183 -> [w194]
              shift-right: [w190] -> w180
              shift-left: w181 -> [w189]
              tunnel: w177 -> [w188]
              tunnel: w176 -> [w187]
              tunnel: w175 -> [w186]
              tunnel: w174 -> [w185]
              stop <- w198 stop-if-true
              # "WiFi版本:\n明核/超敏?"
              # "通信状态机"
              n80 = Unbundle By Name(w194) -> ("探头状态"=w193:T11)
              n81 = case shown="\"禁用\"" w193 {
                tunnel: [w202 w204] -> w192
                tunnel: w191 -> [w202 _]
                frame "正常", Default {
                  # "启用，正常通过"
                }
                frame "禁用" {
                  w204 = enum16{"读指令", "解析实时", "解析限值", "暂停发送", "读取超时"}."暂停发送"  # 暂停
                  # "禁用，则暂停\n并延时"
                  n82 = Wait (ms)(milliseconds to wait=u32 500 ("等待时间（毫秒）")) -> ()  [unwired: 1 out]
                }
              }
              n83 = case shown="\"读指令\", 默认" w192 {
                tunnel: w201 -> [w215 w258 w415 w457 w502]
                tunnel: [w214 w258 w415 w454 w501] -> w200
                tunnel: [w213 w262 w416 w467 w504] -> w199
                tunnel: [_ _ _ "停止" w505] -> w198
                tunnel: [w212 _ _ _ _] -> w197
                tunnel: w196 -> [_ w265 w419 _ _]
                tunnel: w194 -> [w209 w256 w414 w456 w499]
                tunnel: [w211 w261 w413 w455 w494] -> w195
                tunnel: [w210 w260 w412 w466 w503] -> w190
                tunnel: w189 -> [w210 w259 w412 w466 w503]
                tunnel: w188 -> [_ w253 _ w460 _]
                tunnel: w187 -> [w206 w254 _ w449 _]
                tunnel: w186 -> [_ w252 _ _ _]
                tunnel: w185 -> [w205 _ _ _ _]
                frame "读指令", Default {
                  # "只对网络探头 读取来自探头的自动上传指令，超时则错误"
                  n84 = Unbundle By Name(w206) -> ("探头地址(U8)"=w207:u8)
                  n85 = case shown="0" w207 {
                    tunnel: w215 -> [w226 w246]
                    tunnel: [w224 w246] -> w214
                    tunnel: [w222 w247] -> w213
                    tunnel: [w221 _] -> w212
                    tunnel: [w220 _] -> w208
                    tunnel: w205 -> [w216 _]
                    frame 0 {
                      w219 = 9  # 明核9
                      w217 = 10  # 超敏10
                      w225 = 10000  # 超时
                      # "1001版本，10字节数据"
                      # "有些情况下局域网电脑之间通信 在连接后的首次通信时延时较长，之后就好了(不知道为啥)。\n所以，读取超时要留长一点，至少10s。（和连接延时不同）"
                      # "网络探头"
                      n86 = Select(t=w217, s=w216, f=w219) -> (s? t:f=w218:i32)
                      n87 = TCP Read(connection ID=w226, bytes to read=w218, 9:w225) -> (connection ID out=w224:refnum<k5>, data out=w223:string, error out=w220:errorcluster)  [unwired: 2 in]
                      "接收数据" <- w223
                      n88 = case shown="无错误" w220 {
                        tunnel: w223 -> [w232 _]
                        tunnel: [w234 w245] -> w222
                        tunnel: [w232 _] -> w221
                        tunnel: w216 -> [w230 _]
                        frame No Error {
                          w229 = 1  # 明核1
                          w238 = "\t"  # 限值
                          w239 = "\u0003"  # 实时
                          w228 = 2  # 超敏2
                          # "1001版本，2字节地址"
                          # "根据功能码判断是解析什么"
                          n89 = Select(t=w228, s=w230, f=w229) -> (s? t:f=w227:i32)
                          n90 = String Subset(string=w232, offset (0)=w227, length (rest)=1 ("偏移量(0)")) -> (substring=w237:string)
                          n91 = Equal?(x=w239, y=w237) -> (x = y?=w233:bool)
                          n92 = Equal?(x=w237, y=w238) -> (x = y?=w236:bool)
                          n93 = Or(x=w233, y=w236) -> (x .or. y?=w235:bool)
                          n94 = case shown="真" w235 {
                            tunnel: [w240 w241] -> w234
                            tunnel: w233 -> [_ w244]
                            frame False {
                              w240 = enum16{"读指令", "解析实时", "解析限值", "暂停发送", "读取超时"}."暂停发送"  # 暂停发送
                              # "无效功能码，不能解析\n只能直接跳转到 '暂停' 帧"
                            }
                            frame True {
                              w242 = enum16{"读指令", "解析实时", "解析限值", "暂停发送", "读取超时"}."解析限值"  # 限值
                              w243 = enum16{"读指令", "解析实时", "解析限值", "暂停发送", "读取超时"}."解析实时"  # 实时
                              # "有效功能码"
                              n95 = Select(t=w243, s=w244, f=w242) -> (s? t:f=w241:enum16{"读指令", "解析实时", "解析限值", "暂停发送", "读取超时"})
                            }
                          }
                        }
                        frame Error {
                          w245 = enum16{"读指令", "解析实时", "解析限值", "暂停发送", "读取超时"}."暂停发送"  # 暂停
                          # "结束循环，跳出重连"
                        }
                      }
                    }
                    frame 1, Default {
                      w247 = enum16{"读指令", "解析实时", "解析限值", "暂停发送", "读取超时"}."解析实时"  # 实时
                      # "串口版探头不会自动上报报警值,\n所以只需要读实时数据"
                      # "串口探头, (无错误, 解析实时,空数据)"
                    }
                  }
                  n96 = local write "通信错误"(w208) -> ()
                  n97 = in-place {
                    in-place-border: w208 -> [w251]
                    w250 = 探头状态."离线"  # 离线
                    n98 = in-place-cluster #4(w209) -> ("探头状态"=w248:T11)
                    n99 = Select(t=w250, s=w251, f=w248) -> (s? t:f=w249:T11)
                    n100 = in-place-cluster #4("探头状态"=w249) -> (w211:T8)
                  }
                }
                frame "解析实时" {
                  w262 = enum16{"读指令", "解析实时", "解析限值", "暂停发送", "读取超时"}."暂停发送"  # 暂停
                  # "( 仅串口探头在此发送请求) 同时 判断报警状态 , 计算和更新累积剂量"
                  n101 = Unbundle By Name(w254) -> ("探头地址(U8)"=w257:u8)
                  n102 = case shown="0" w257 {
                    tunnel: w265 -> [w269 _]
                    tunnel: [w268 w277] -> w264
                    tunnel: [w267 w278] -> w263
                    tunnel: w254 -> [_ w280]
                    tunnel: w256 -> [w266 w276]
                    tunnel: [w266 w275] -> w255
                    tunnel: w252 -> [_ w270]
                    frame 0 {
                      # "网络探头, 1001 协议"
                      n103 = call "测量数据解析-1001.vi"("完整输入"=w269) -> ("CRC？"=w268:bool, "测量值"=w267:dbl)  [unwired: 8 in, 1 out]
                    }
                    frame 1, Default {
                      w281 = 串口动作类型."读测量值"  # 读测量值
                      # "串口探头,"
                      n104 = Bundle By Name(cluster=T20 {"串口动作类型"=enum."读测量值", "串口配置"={"COM口"="", "波特率"=enum."9600", "探头地址(U8)"=0}, "数据输入"=variant} ("串口模块输入"), "串口动作类型"=w281, "串口配置"=w280) -> (w284:T20)
                      n105 = call "TOP-串口通信模块.vi"("串口模块输入"=w284) -> ("error out"=w274:errorcluster, "数据输出"=w285:variant)  [unwired: 9 in]
                      n106 = case shown="错误" w274 {
                        selector: w274 -> [_ w290]
                        tunnel: w276 -> [w286 w295]
                        tunnel: [w286 w294] -> w275
                        tunnel: [_ w293] -> w273
                        tunnel: [_ w289] -> w271
                        tunnel: w270 -> [_ w287]
                        frame No Error {
                        }
                        frame Error {
                          # "丢包几次之后认为掉线"
                          n107 = Increment(x="串口丢包次数") -> (x+1=w293:i32)
                          n108 = Greater?(x=w293, y=w287) -> (0:w291:bool)
                          n109 = Select(t=w290, s=w291, f=errorcluster {"status"=FALSE, "code"=0, "source"=""} ("通信错误")) -> (s? t:f=w289:errorcluster)
                          n110 = in-place {
                            in-place-border: w291 -> [w299]
                            w297 = 探头状态."离线"  # 离线
                            n111 = in-place-cluster #5(w295) -> ("探头状态"=w298:T11)
                            n112 = Select(t=w297, s=w299, f=w298) -> (s? t:f=w296:T11)
                            n113 = in-place-cluster #5("探头状态"=w296) -> (w294:T8)
                          }
                        }
                      }
                      n114 = Variant To Data(type=T24 {"测量值"=0.0, "CRC"=FALSE, "接收指令"=""} ("测量值读取"), Variant=w285) -> (data=w279:T24)  [unwired: 1 in, 1 out]
                      n115 = Unbundle By Name(w279) -> ("接收指令"=w272:string, "CRC"=w277:bool, "测量值"=w278:dbl)
                      n116 = local write "串口丢包次数"(w273) -> ()
                      n117 = local write "通信错误"(w271) -> ()
                      n118 = local write "接收数据"(w272) -> ()
                    }
                  }
                  n119 = case shown="真" w264 {
                    tunnel: w263 -> [_ w323]
                    tunnel: w255 -> [w301 w310]
                    tunnel: [w301 w311] -> w261
                    tunnel: [w300 w313] -> w260
                    tunnel: w259 -> [w300 w312]
                    tunnel: w258 -> [_ w309]
                    tunnel: w254 -> [_ w303]
                    tunnel: w253 -> [_ w302]
                    frame False {
                      # "数据不完整"
                    }
                    frame True {
                      w306 = 探头状态."一级报警"  # 一级
                      w305 = 探头状态."二级报警"  # 二级
                      w322 = 探头状态."一级报警"  # 一级
                      w320 = 探头状态."二级报警"  # 二级
                      w325 = cluster{"时间":timestamp, "数值":dbl} {"时间"=timestamp(0 s since 1904-01-01), "数值"=0.0}  # 测量值
                      # "数据完整有效"
                      n120 = Get Date/Time In Seconds() -> (seconds since 1Jan1904=w324:timestamp)
                      n121 = Bundle By Name(cluster=w325, "数值"=w323, "时间"=w324) -> (w314:cluster{"时间":timestamp, "数值":dbl})
                      n122 = in-place {
                        in-place-border: w314 -> [w378]
                        in-place-border: w323 -> [w365]
                        in-place-border: [w381] -> w321
                        in-place-border: [w380] -> w307
                        in-place-border: w309 -> [w362]
                        in-place-border: w303 -> [w356]
                        in-place-border: w302 -> [w355]
                        w370 = enum16{"一级限值", "二级限值"}."一级限值"  # 一级
                        w374 = T25 {"探头地址与信息"={"网络地址"="", "名称"="", "备注"="", "累积剂量"=0.0, "累积限值"=0.0, "硬件剂量率限值"=enum."一级限值", "剂量率限值1"=0.0, "剂量率限值2"=0.0, "报警方式"=enum."常报警"}, "测量值"={"时间"=timestamp(0 s since 1904-01-01), "数值"=0.0}, "累积记录"={"起始时间"=timestamp(0 s since 1904-01-01), "结束时间"=timestamp(0 s since 1904-01-01), "累积剂量"=0.0}}
                        n123 = in-place-cluster #6(w310) -> ("报警方式"=w364:T13, "限值"=w385:T10, "探头状态"=w381:T11, "累积记录"=w377:T12, "探头地址与信息"=w358:T5)  [unwired: 1 out]
                        n124 = Bundle By Name(cluster=w374, "探头地址与信息"=w358, "测量值"=w378, "累积记录"=w377) -> (w376:T25)
                        n125 = Unbundle By Name(w385) -> ("探头限值"=w369:T6, "限值1"=w367:dbl, "限值2"=w366:dbl)
                        n126 = Greater? "二级？"(x=w365, y=w366) -> (0:w384:bool)
                        n127 = Greater? "一级？"(x=w365, y=w367) -> (0:w383:bool)
                        n128 = Equal?(x=w370, y=w369) -> (x = y?=w368:bool)
                        n129 = Bundle By Name(cluster=T22 {"动作类型"=enum."DB-文件初始化+连接", "输入数据"=variant} ("指令与数据"), "动作类型"=DB动作类型."数据-写改累积记录+改累积剂量", "输入数据"=w376) -> (w359:T22)
                        n130 = And "二级报警？"(x=w383, y=w384) -> (x .and. y?=w382:bool)
                        n131 = Select "硬件限值"(t=w367, s=w368, f=w366) -> (s? t:f=w360:dbl)
                        n132 = Greater Or Equal? "硬件未报警？"(x=w360, y=w365) -> (x >= y?=w361:bool)
                        n133 = call "TOP-累积剂量数据管理.vi"("DB动作集"=w359) -> ("输出数据"=w375:variant)  [unwired: 9 in, 1 out]
                        n134 = Variant To Data(type=w374, Variant=w375) -> (data=w373:T25)  [unwired: 1 in, 1 out]
                        n135 = call "报警方式处理模块-网络版.vi"("串口配置"=w356, "连接ID"=w362, "硬件限值"=w360, "硬件未报警？"=w361, "报警方式 i"=w364) -> ("报警方式 o"=w363:T26)  [unwired: 5 in, 1 out]
                        n136 = Unbundle By Name(w373) -> ("累积记录"=w372:T12, "探头地址与信息"=w371:T5)
                        n137 = case shown="假" w382 {
                          tunnel: w383 -> [w397 _]
                          tunnel: [w395 w410] -> w380
                          tunnel: w373 -> [w387 _]
                          tunnel: w358 -> [w388 _]
                          tunnel: w355 -> [w386 _]
                          frame False {
                            w391 = 探头状态."累积报警"  # 累积报警
                            w390 = 探头状态."正常"  # 正常
                            w396 = 探头状态."一级报警"  # 一级
                            # "非 二级报警"
                            n138 = Unbundle By Name(w387) -> ("探头地址与信息.累积剂量"=w393:dbl, "探头地址与信息.累积限值"=w394:dbl)
                            n139 = Greater?(x=w393, y=w394) -> (0:w389:bool)
                            n140 = Select "累积报警？"(t=w391, s=w389, f=w390) -> (s? t:f=w392:T11)
                            n141 = Select "一级报警？"(t=w396, s=w397, f=w392) -> (s? t:f=w395:T11)
                            n142 = case shown="真" w389 {
                              tunnel: w388 -> [_ w403]
                              tunnel: w387 -> [_ w399]
                              tunnel: w386 -> [_ w398]
                              frame False {
                                # "非累积报警"
                              }
                              frame True {
                                # "现在发生累积报警"
                                n143 = Unbundle By Name(w403) -> ("累积剂量"=w402:dbl, "累积限值"=w401:dbl)
                                n144 = Greater?(x=w402, y=w401) -> (0:w400:bool)
                                n145 = case shown="假" w400 {
                                tunnel: w399 -> [w405 _]
                                tunnel: w398 -> [w404 _]
                                frame False {
                                # "原没累积报警，生成"
                                n146 = stacked-sequence {
                                tunnel: w405 -> [w407 _]
                                tunnel: w404 -> [_ w408]
                                frame #0 {
                                # "生成文件"
                                n147 = Unbundle By Name(w407) -> ("探头地址与信息"=w406:T5)
                                n148 = call "生成-累积剂量报警记录数据文件-网络版.vi"("探测器信息"=w406) -> ()  [unwired: 11 in]
                                }
                                frame #1 {
                                # "刷新列表"
                                n149 = property on="新记录刷新" class="Ctl"(reference=w408, "Val(Sgnl)"=TRUE) -> ()  [unwired: 1 in, 2 out]
                                }
                                }
                                }
                                frame True {
                                }
                                }
                              }
                            }
                          }
                          frame True {
                            w410 = 探头状态."二级报警"  # 二级
                            # "二级报警"
                          }
                        }
                        n150 = in-place-cluster #6("报警方式"=w363, "测量值"=w378, "限值"=w385, "探头状态"=w380, "累积记录"=w372, "探头地址与信息"=w371) -> (w311:T8)
                      }
                      n151 = Equal?(x=w321, y=w320) -> (x = y?=w318:bool)
                      n152 = Equal?(x=w321, y=w322) -> (x = y?=w319:bool)
                      n153 = Or "原：报警？"(x=w319, y=w318) -> (x .or. y?=w317:bool)
                      n154 = Not Equal?(x=w307, y=w306) -> (x != y?=w316:bool)
                      n155 = Not Equal?(x=w307, y=w305) -> (x != y?=w304:bool)
                      n156 = And "现正常？"(x=w316, y=w304) -> (x .and. y?=w308:bool)
                      n157 = And "报警刚结束?"(x=w308, y=w317) -> (x .and. y?=w315:bool)
                      n158 = case shown="假" w308 {
                        tunnel: w315 -> [_ w341]
                        tunnel: w312 -> [w330 w339]
                        tunnel: [w328 w340] -> w313
                        tunnel: w311 -> [w334 _]
                        frame False {
                          # "现：发生报警，缓存"
                          n159 = Unbundle By Name(w334) -> ("探头地址与信息.名称"=w331:string, "测量值"=w329:T9)
                          n160 = call "动态时值缓存指数压缩.vi"("新数据"=w329, "缓存数据"=w330) -> ("缓存数据 o"=w328:T2)  [unwired: 9 in]
                          n161 = Unbundle By Name(w328) -> ("压缩等级数量"=w327:i32[])
                          n162 = Add Array Elements(numeric array=w327) -> (sum=w326:i32)
                          n163 = Equal?(x=10, y=w326) -> (x = y?=w332:bool)
                          n164 = disable-structure shown="禁用" {
                            disable-tunnel: w332 -> [w336 _]
                            disable-tunnel: w331 -> [w335 _]
                            frame Disabled {
                              n165 = case shown="真" w336 {
                                tunnel: w335 -> [_ w337]
                                frame False {
                                }
                                frame True {
                                # "10s短信报警"
                                n166 = call "短信通知-发送.vi"("探头名称"=w337) -> ()  [unwired: 11 in]
                                }
                              }
                            }
                            frame Enabled {
                            }
                          }
                        }
                        frame True {
                          # "现：未报警,  防抖动"
                          n167 = case shown="假" w341 {
                            tunnel: [w343 w353] -> w340
                            tunnel: w339 -> [w342 w353]
                            tunnel: [w345 w354] -> w338
                            frame False {
                              # "原：未报警，正常, 额外检查5防抖"
                              n168 = case shown="0" "报警缓存防抖计次" {
                                selector: "报警缓存防抖计次" -> [_ w348 _]
                                tunnel: [_ w347 _] -> w345
                                tunnel: [_ w346 _] -> w343
                                tunnel: w342 -> [_ w346 w349]
                                frame 0 {
                                # "=0, 说明现在没有"
                                }
                                frame Default {
                                # "防抖中, 防抖计次"
                                n169 = Increment(x=w348) -> (x+1=w347:i32)
                                }
                                frame 6.. {
                                w351 = T1 {"新记录？"=TRUE, "缓存数据"={"时间"=[], "数值"=[], "压缩等级数量"=[], "最大值"={"时间"=timestamp(0 s since 1904-01-01), "数值"=0.0}, "起始点"={"时间"=timestamp(0 s since 1904-01-01), "数值"=0.0}, "容量限值"=0, "报警累积"=0.0}}  # 缓存结果
                                w350 = TRUE  # T
                                # "防抖已过, 确认生成记录, 关闭防抖"
                                n170 = Bundle By Name(cluster=w351, "新记录？"=w350, "缓存数据"=w349) -> (w352:T1)
                                n171 = local write "缓存结果"(w352) -> ()
                                }
                              }
                            }
                            frame True {
                              w354 = 1  # 1: 开始防抖
                              # "原：报警，报警结束, 防抖开始"
                            }
                          }
                          n172 = local write "报警缓存防抖计次"(w338) -> ()
                        }
                      }
                    }
                  }
                }
                frame "解析限值" {
                  w416 = enum16{"读指令", "解析实时", "解析限值", "暂停发送", "读取超时"}."暂停发送"  # 暂停
                  # "串口探头不会执行到这里"
                  # "报警限值回复，设置成功则状态栏提示"
                  n173 = call "报警设置-回执解析.vi"("完整输入"=w419) -> ("有效数据？"=w418:bool, "探头号"=w411:u16, "限值"=w417:dbl)  [unwired: 8 in]
                  n174 = case shown="真" w418 {
                    tunnel: w417 -> [w424 w436]
                    tunnel: w414 -> [w421 w431]
                    tunnel: [w420 w431] -> w413
                    tunnel: w411 -> [_ _]
                    frame False {
                      # "无效数据"
                      n175 = Equal?(x=inf, y=w424) -> (x = y?=w422:bool)
                      n176 = case shown="真" w422 {
                        tunnel: w421 -> [w425 w427]
                        tunnel: [w425 w426] -> w420
                        frame False {
                        }
                        frame True {
                          # "返回报警限值为 正无穷 ， 说明硬件静音了"
                          n177 = in-place {
                            n178 = in-place-cluster #7(w427) -> ()  [unwired: 1 out]
                            n179 = in-place-cluster #7("报警方式.报警中？"=FALSE) -> (w426:T8)
                          }
                        }
                      }
                    }
                    frame True {
                      w435 = 1000.0 ("y")
                      # "有效数据, 提示"
                      n180 = Greater Or Equal?(x=w436, y=w435) -> (x >= y?=w437:bool)
                      n181 = case shown="假" w437 {
                        tunnel: [w439 w441] -> w433
                        tunnel: w436 -> [w439 w442]
                        tunnel: ["μSv/h" ("单位") "mSv/h" ("单位")] -> w432
                        tunnel: w435 -> [_ w440]
                        frame False {
                          # "uSv/h"
                        }
                        frame True {
                          # "mSv/h"
                          n182 = Divide(x=w442, y=w440) -> (x/y=w441:dbl)
                        }
                      }
                      n183 = Unbundle By Name(w431) -> ("探头地址与信息.名称"=w429:string)
                      n184 = call "创建文本"("探头名称"=w429, "限值"=w433, "单位"=w432) -> ("Result"=w434:string)  [unwired: 11 in, 1 out]
                      n185 = call "状态栏-插入状态信息-35点监测专用.vi"("消息内容"=w434, "状态类型"=enum16{"全部", "报警", "通信", "设置"}."设置") -> ()  [unwired: 10 in]
                    }
                  }
                }
                frame "暂停发送" {
                  w452 = enum16{"连接模式", "离线模式"}."连接模式"  # 连接模式
                  w469 = enum16{"读指令", "解析实时", "解析限值", "暂停发送", "读取超时"}."读取超时"  # 结束循环
                  w468 = enum16{"读指令", "解析实时", "解析限值", "暂停发送", "读取超时"}."读指令"  # 读指令
                  # "串口通信要主动延时 1s"
                  # "暂停发送，判断是否有变动，更新“探头属性”，下一帧为“读数据”"
                  n186 = Unbundle By Name(w449) -> ("探头地址(U8)"=w448:u8)
                  n187 = case shown="错误" "通信错误" {
                    tunnel: "缓存结果" -> [w470 w474]
                    tunnel: [w470 w471] -> w462
                    frame No Error {
                      # "正常执行"
                    }
                    frame Error {
                      # "掉线，但有未保存缓存\n直接生成记录"
                      n188 = Unbundle By Name(w474) -> ("缓存数据.数值"=w475:dbl[])
                      n189 = Empty Array? "空？"(array=w475) -> (empty?=w473:bool)
                      n190 = Not "非"(x=w473) -> (.not. x?=w472:bool)
                      n191 = Bundle By Name(cluster=w474, "新记录？"=w472) -> (w471:T1)
                    }
                  }
                  n192 = Not Equal To 0?(x=w448) -> (x != 0?=w447:bool)
                  n193 = call "改动项处理模块.vi"("执行模式"=w452, "改动项 i"="改动项", "串口配置"=w449, "探头属性 i"=w456, "TCP ID i"=w457) -> ("error out"=w453:errorcluster, "探头属性 o"=w455:T8, "TCP ID o"=w454:refnum<k5>, "改动项复位 o"=w458:T3)  [unwired: 3 in]
                  n194 = local write "改动项"(w458) -> ()
                  n195 = Select(t=u32 1000, s=w447, f=u32 0) -> (s? t:f=w444:u32)
                  n196 = local write "探头属性"(w455) -> ()
                  n197 = Unbundle By Name(w462) -> ("新记录？"=w463:bool)
                  n198 = call "Stall Data Flow.vim"("value in"=w453, "milliseconds to wait"=w444) -> ("value out"=w450:errorcluster)  [unwired: 1 out]
                  n199 = case shown="真" w463 {
                    tunnel: w462 -> [_ w478]
                    tunnel: w456 -> [_ w477]
                    tunnel: w460 -> [_ w476]
                    frame False {
                      # "没有新缓存"
                    }
                    frame True {
                      # "产生新缓存记录"
                      n200 = stacked-sequence {
                        tunnel: w478 -> [w482 _]
                        tunnel: w477 -> [w480 _]
                        tunnel: w476 -> [_ w488]
                        frame #0 {
                          # "生成缓存文件"
                          n201 = Unbundle By Name(w480) -> ("探头地址与信息"=w479:T5)
                          n202 = Unbundle By Name(w482) -> ("缓存数据"=w481:T2)
                          n203 = call "生成-剂量率报警记录数据文件-网络版.vi"("缓存绘图数据"=w481, "探测器信息"=w479) -> ()  [unwired: 10 in]
                        }
                        frame #1 {
                          w485 = T1 {"新记录？"=FALSE, "缓存数据"={"时间"=[], "数值"=[], "压缩等级数量"=[], "最大值"={"时间"=timestamp(0 s since 1904-01-01), "数值"=0.0}, "起始点"={"时间"=timestamp(0 s since 1904-01-01), "数值"=0.0}, "容量限值"=0, "报警累积"=0.0}}  # 缓存结果
                          # "清除缓存数据，通知主VI刷新"
                          n204 = property on="新记录刷新" class="Ctl"(reference=w488, "Val(Sgnl)"=TRUE) -> ()  [unwired: 1 in, 2 out]
                          n205 = Bundle By Name(cluster=w485, "新记录？"=FALSE, "缓存数据"=T2 {"时间"=[], "数值"=[], "压缩等级数量"=[], "最大值"={"时间"=timestamp(0 s since 1904-01-01), "数值"=0.0}, "起始点"={"时间"=timestamp(0 s since 1904-01-01), "数值"=0.0}, "容量限值"=0, "报警累积"=0.0}) -> (w486:T1)
                          n206 = local write "缓存结果"(w486) -> ()
                        }
                      }
                    }
                  }
                  n207 = case shown="真" "停止" {
                    tunnel: w454 -> [_ w490]
                    frame False {
                    }
                    frame True {
                      # "外部给出关闭信号"
                      n208 = TCP Close Connection(connection ID=w490) -> (error out=w489:errorcluster)  [unwired: 2 in, 1 out]
                      n209 = call <vilib>:"Clear Errors.vi"("error in (no error)"=w489) -> ()  [unwired: 5 in, 2 out]
                    }
                  }
                  n210 = Merge Errors(w450, "通信错误") -> (w465:errorcluster)
                  n211 = Select(t=w469, s=w465, f=w468) -> (s? t:f=w467:enum16{"读指令", "解析实时", "解析限值", "暂停发送", "读取超时"})
                }
                frame "读取超时" {
                  w491 = 0.0  # 校准值
                  w495 = DB动作类型."设备-累积校准"  # 累积校准
                  w504 = enum16{"读指令", "解析实时", "解析限值", "暂停发送", "读取超时"}."读指令"  # 读指令
                  w505 = TRUE  # T
                  # "关闭连接，结束循环，结束此次累积 , 校准同步总累积，跳出重连"
                  n212 = TCP Close Connection(connection ID=w502) -> (connection ID out=w501:refnum<k5>, error out=w500:errorcluster)  [unwired: 2 in]
                  n213 = call <vilib>:"Clear Errors.vi"("error in (no error)"=w500) -> ()  [unwired: 5 in, 2 out]
                  n214 = Unbundle By Name(w499) -> ("探头地址与信息.名称"=w496:string)
                  n215 = Bundle By Name(cluster=T22 {"动作类型"=enum."DB-文件初始化+连接", "输入数据"=variant} ("DB动作集"), "动作类型"=w495, "输入数据"=w496) -> (w497:T22)
                  n216 = call "TOP-累积剂量数据管理.vi"("DB动作集"=w497) -> ("输出数据"=w493:variant)  [unwired: 9 in, 1 out]
                  n217 = Variant To Data(type=w491, Variant=w493) -> (data=w492:dbl)  [unwired: 1 in, 1 out]
                  n218 = Bundle By Name(cluster=w499, "探头地址与信息.累积剂量"=w492) -> (w494:T8)
                }
              }
            }
          }
          frame Error {
            w514 = enum16{"连接模式", "离线模式"}."离线模式"  # 离线模式
            # "串口通信, 掉线时应该加个延时, 不然发指令频率太快"
            n219 = Unbundle By Name(w511) -> ("探头地址(U8)"=w510:u8)
            n220 = Not Equal To 0?(x=w510) -> (x != 0?=w509:bool)
            n221 = Select(t=u32 500 ("等待时间（毫秒）"), s=w509, f=u32 0 ("等待时间（毫秒）")) -> (s? t:f=w506:u32)
            n222 = TCP Close Connection(connection ID=w515) -> (connection ID out=w518:refnum<k5>, error out=w519:errorcluster)  [unwired: 2 in]
            n223 = Wait (ms)(milliseconds to wait=w506) -> ()  [unwired: 1 out]
            n224 = call <vilib>:"Clear Errors.vi"("error in (no error)"=w519) -> ()  [unwired: 5 in, 2 out]
            n225 = local read "改动项"() -> (w517:T3)
            n226 = call "改动项处理模块.vi"("执行模式"=w514, "改动项 i"=w517, "串口配置"=w511, "探头属性 i"=w513, "TCP ID i"=w515) -> ("探头属性 o"=w512:T8, "改动项复位 o"=w516:T3)  [unwired: 3 in, 2 out]
            n227 = local write "改动项"(w516) -> ()
            n228 = local write "探头属性"(w512) -> ()
          }
        }
      }
    }
    n229 = local write "报警缓存防抖计次"(w30) -> ()
    n230 = local read "停止"() -> (w45:bool)
  }
  n231 = case shown="假" w1 {
    frame False {
      # "明核/速核的 wifi版"
      n232 = node-c288() -> (w522:T27)  [unwired: 4 in]
      n233 = timed-loop {
        timing: w522 -> [_]
        timing-out: [_] -> w521
        i -> [w524]
        stop <- w523 stop-if-true
        w526 = "\u0001\u0003\u0000€ú\u0000\u0006‚"  # 读实时
        # "发送指令读实时数据"
        n234 = node-c288() -> ()  [unwired: 1 in, 1 out]
        n235 = local read "TCP连接ID"() -> (w527:refnum<k5>)
        n236 = local read "停止"() -> (w523:bool)
        n237 = TCP Write(connection ID=w527, data in=w526, 9:900 ("超时毫秒(25000)")) -> (error out=w525:errorcluster)  [unwired: 1 in, 2 out]
        n238 = local write "通信错误"(w525) -> ()
        n239 = node-c288() -> ()  [unwired: 1 in, 1 out]
        "循环次数" <- w524
      }
      n240 = node-c288(w521) -> ()  [unwired: 1 out]
    }
    frame True {
    }
  }
